vi "svfa_Tone Estimation Subroutine G(f) (first derivative).vi"   [LabVIEW 2017]
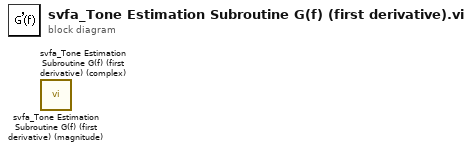
[diagram p0: block diagram]
diagram:
  n1 = call <vilib>:"svfa_Tone Estimation Subroutine G(f) (first derivative) (magnitude).vi"() -> ()  [unwired: 4 in, 1 out]
  n2 = call <vilib>:"svfa_Tone Estimation Subroutine G(f) (first derivative) (complex).vi"() -> ()  [unwired: 4 in, 1 out]
